vi "Security_Code.vi"() -> ()   [LabVIEW 2022 SP3]
uses:
  <vilib>/numeric/Random Number (Range) I64.vi
  <vilib>/numeric/sub_Random U32.vi
panel:
  out "?":bool
  out "?":dbl
  out "?":dbl
  in  "?":dbl
  out "?":bool
  out "?":dbl
  out "?":dbl
  in  "?":dbl
  out "?":bool
  out "?":dbl
  out "?":dbl
  in  "?":dbl
  out "?":bool
  out "?":dbl
  out "?":dbl
  in  "?":dbl
  # "Security_Code:"
  # "Enter a security code with numbers 0-9"
  # "Security Code"
  # "Guessed Number"
  # "Number of Attempts"
  # "Lock"
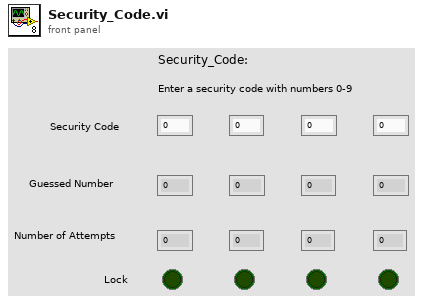
[diagram p1: front panel]
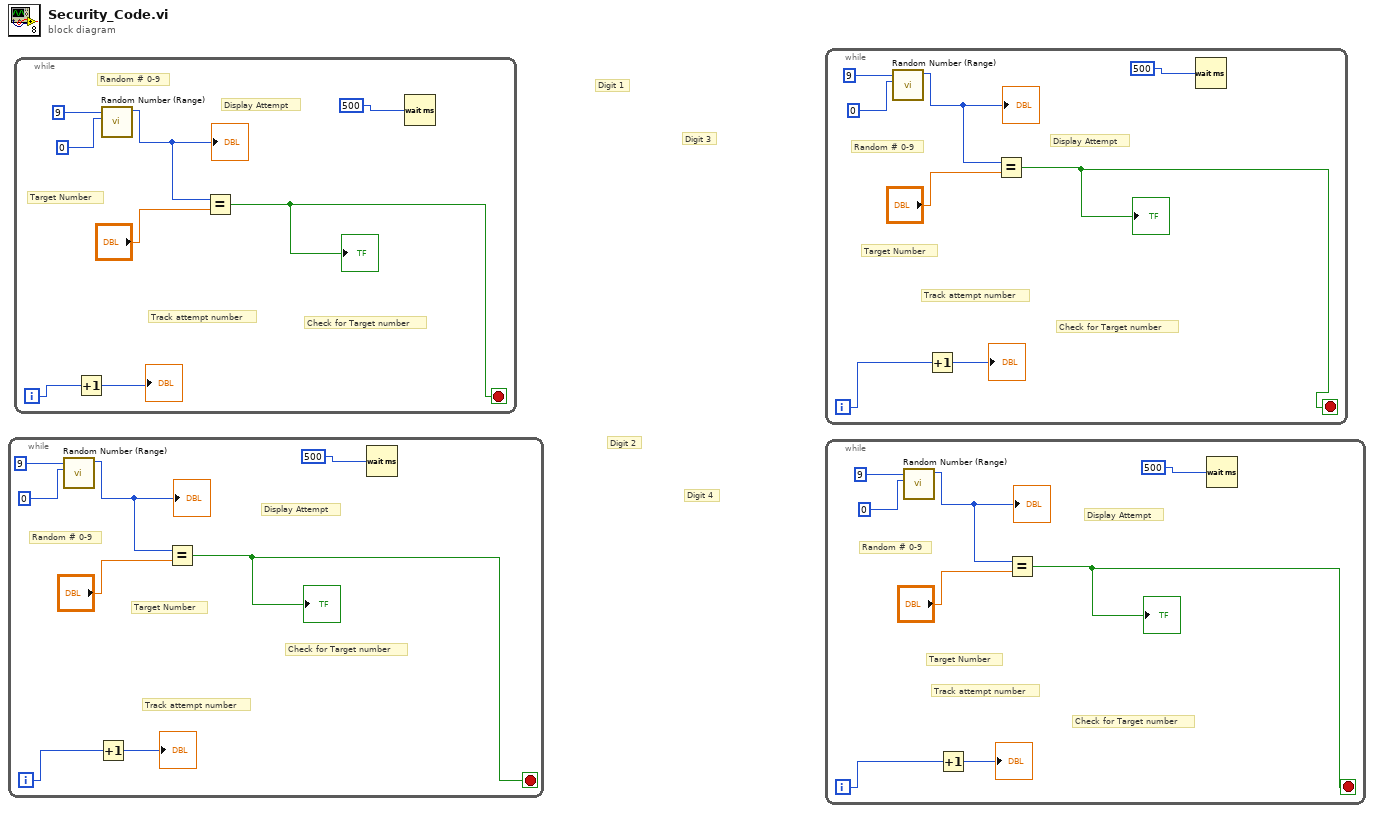
[diagram p0: block diagram]
diagram:
  # "Digit 4"
  # "Digit 3"
  # "Digit 2"
  # "Digit 1"
  n1 = while {
    i -> [w1]
    stop <- w3 stop-if-true
    # "Check for Target number"
    # "Target Number"
    # "Random # 0-9"
    # "Display Attempt"
    # "Track attempt number"
    n2 = call-poly <vilib>:"Random Number (Range).vi"("lower bound (-100)"=0, "upper bound (100)"=9) -> ("number"=w7:i64)  [unwired: 9 in]
    "?" <- w7
    n3 = Increment(x=w1) -> (x+1=→"?":i32)
    n4 = Equal?(x=w7, y="?") -> (x = y?=w3:bool)
    "?" <- w3
    n5 = Wait (ms)(milliseconds to wait=500) -> ()  [unwired: 1 out]
  }
  n6 = while {
    i -> [w14]
    stop <- w9 stop-if-true
    # "Track attempt number"
    # "Check for Target number"
    # "Target Number"
    # "Display Attempt"
    # "Random # 0-9"
    n7 = Increment(x=w14) -> (x+1=→"?":i32)
    n8 = call-poly <vilib>:"Random Number (Range).vi"("lower bound (-100)"=0, "upper bound (100)"=9) -> ("number"=w12:i64)  [unwired: 9 in]
    "?" <- w12
    n9 = Equal?(x=w12, y="?") -> (x = y?=w9:bool)
    "?" <- w9
    n10 = Wait (ms)(milliseconds to wait=500) -> ()  [unwired: 1 out]
  }
  n11 = while {
    i -> [w17]
    stop <- w18 stop-if-true
    # "Check for Target number"
    # "Target Number"
    # "Random # 0-9"
    # "Display Attempt"
    # "Track attempt number"
    n12 = call-poly <vilib>:"Random Number (Range).vi"("lower bound (-100)"=0, "upper bound (100)"=9) -> ("number"=w23:i64)  [unwired: 9 in]
    "?" <- w23
    n13 = Increment(x=w17) -> (x+1=→"?":i32)
    n14 = Equal?(x=w23, y="?") -> (x = y?=w18:bool)
    "?" <- w18
    n15 = Wait (ms)(milliseconds to wait=500) -> ()  [unwired: 1 out]
  }
  n16 = while {
    i -> [w25]
    stop <- w26 stop-if-true
    # "Check for Target number"
    # "Target Number"
    # "Random # 0-9"
    # "Display Attempt"
    # "Track attempt number"
    n17 = call-poly <vilib>:"Random Number (Range).vi"("lower bound (-100)"=0, "upper bound (100)"=9) -> ("number"=w31:i64)  [unwired: 9 in]
    "?" <- w31
    n18 = Increment(x=w25) -> (x+1=→"?":i32)
    n19 = Equal?(x=w31, y="?") -> (x = y?=w26:bool)
    "?" <- w26
    n20 = Wait (ms)(milliseconds to wait=500) -> ()  [unwired: 1 out]
  }
